vi "Set JSON Scalar.vi"(8 "error in (no error)":errorcluster, 9 "Set as a JSON string (F)":bool, 10 "LabVIEW Text":string, 11 "JSON Scalar in":refnum<class "JSON Scalar.lvclass">) -> (0 "error out":errorcluster, 3 "JSON Scalar out":refnum<class "JSON Scalar.lvclass">)   [LabVIEW 2011, in "JSON Scalar.lvclass"]
doc: "Stores a <b>String</b> as a <b>JSON Scalar</b>.\nUse <b>Set as a JSON string</b> to indicate it's a formatted string.\n\nCopyright 2012 James David Powell, Shaun Rumbell and Ton Plomp\nMore information on http://lavag.org/topic/16217-cr-json-labview"
uses:
  JSON Scalar.lvclass
  JSON Scalar.lvclass/JSON Scalar.ctl
  JSON Value/JSON Value.lvclass
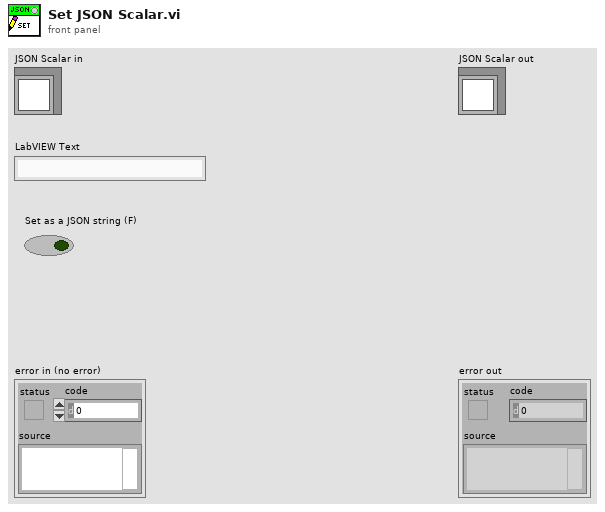
[diagram p1: front panel]
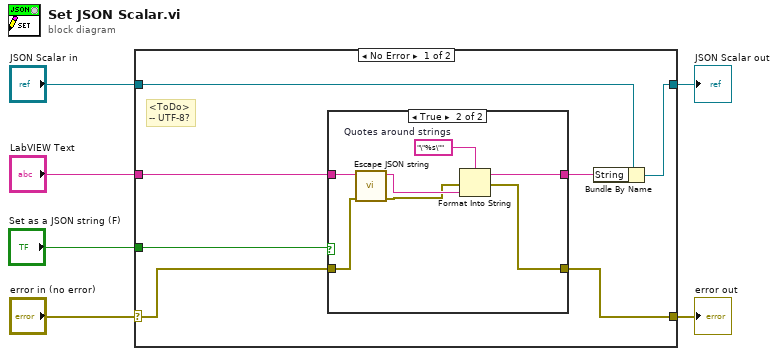
[diagram p0: block diagram]
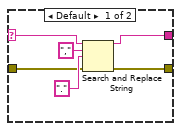
[diagram p3: hidden frame]
diagram:
  n1 = case shown="No Error" "error in (no error)" {
    selector: "error in (no error)" -> [w8 w33]
    tunnel: [w7 w33] -> w5
    tunnel: [w12 w34] -> w3
    tunnel: "JSON Scalar in" -> [w13 w34]
    tunnel: "LabVIEW Text" -> [w10 _]
    tunnel: "Set as a JSON string (F)" -> [w9 _]
    frame No Error {
      # "<ToDo>\n-- UTF-8?"
      n2 = case shown="True" w9 {
        tunnel: [w16 w31] -> w11
        tunnel: w10 -> [w17 w29]
        tunnel: w8 -> [w15 w27]
        tunnel: [w14 w30] -> w7
        frame False {
          n3 = case shown="\"NaN\"" w17 {
            selector: w17 -> [w21 w25]
            tunnel: [w20 w25] -> w16
            tunnel: w15 -> [w19 w24]
            tunnel: [w18 w24] -> w14
            frame Default {
              n4 = Search and Replace String(input string=w21, search string=",", replace string="." ("replace string (\"\")"), error in=w19) -> (result string=w20:string, error out=w18:errorcluster)  [unwired: 4 in, 2 out]
            }
            frame "NaN" {
              # "<ToDo>"
            }
          }
        }
        frame True {
          w32 = "\"%s\""  # Quotes around strings
          n5 = call "Escape JSON string.vi"("error in (no error)"=w27, "Text (unscaped)"=w29) -> ("error out"=w26:errorcluster, "Text (escaped)"=w28:string)  [unwired: 8 in]
          n6 = Format Into String(format string=w32, error in=w26, w28) -> (resulting string=w31:string, error out=w30:errorcluster)  [unwired: 1 in]
        }
      }
      n7 = Bundle By Name(cluster=w13, "String"=w11) -> (w12:refnum<class "JSON Scalar.lvclass">)
    }
    frame Error {
    }
  }
  "error out" <- w5
  "JSON Scalar out" <- w3
